vi "U3 DAC Function Generator.vi"() -> ()   [LabVIEW 2010]
panel:
  out "Error":string
  in  "Min Voltage":dbl=0.5 min=0.0 max=5.0 step=0.1 format="%.2f"
  in  "Stop":bool
  # "SMT Signal Cluster (complexl).ctlUpdates DAC0 at the specified update interval in order to build time series waveforms.  The\nupdate interval is set to 20 ms by default, but can be set lower based on the execution times\ndiscussed in Section 3.1 of the U3 User's Guide.  Uses the first found U3.\n\nWith a software timed application such as this, you might be able to reduce timing jitter (caused\nby the operating system) by increasing the priority of this process (labview.exe) in Windows\nTask Manager."
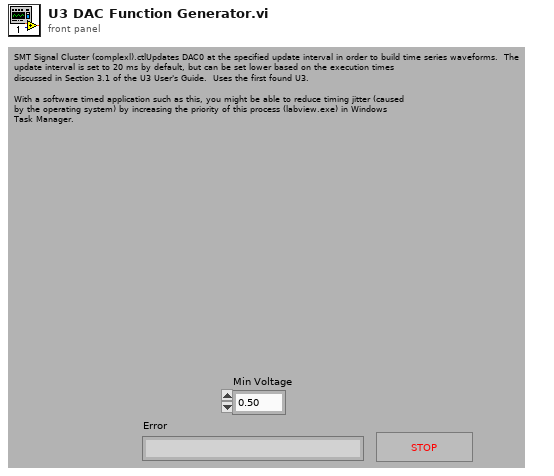
[diagram p1: front panel]
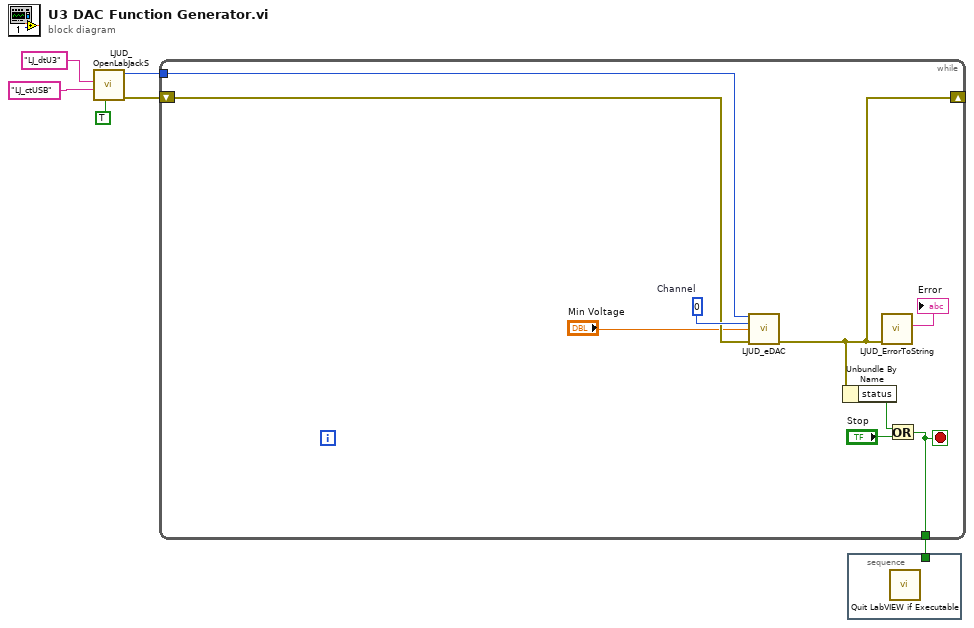
[diagram p0: block diagram]
diagram:
  n1 = call "LJUD_OpenLabJackS.vi"("FirstFound"=TRUE, "ConnectionType"="LJ_ctUSB", "DeviceType"="LJ_dtU3") -> ("error out"=w2:errorcluster, "Handle"=w1:i32)  [unwired: 6 in, 1 out]
  n2 = while {
    tunnel: w1 -> [w8]
    shift-left: w2 -> [w10]
    shift-right: [w9] -> _
    tunnel: [w12] -> w6
    stop <- w12 stop-if-true
    w11 = 0  # Channel
    n3 = call "LJUD_eDAC.vi"("Handle In"=w8, "Channel"=w11, "Voltage"="Min Voltage", "error in"=w10) -> ("error out"=w9:errorcluster)  [unwired: 10 in, 1 out]
    n4 = Unbundle By Name(w9) -> ("status"=w13:bool)
    n5 = call "LJUD_ErrorToString.vi"("error in"=w9) -> ("String"=→"Error":string)  [unwired: 10 in]
    n6 = Or(x=w13, y="Stop") -> (x .or. y?=w12:bool)
  }
  n7 = stacked-sequence {
    tunnel: w6 -> [_]
    frame #0 {
      n8 = call "Quit LabVIEW if Executable.vi"() -> ()  [unwired: 1 in]
    }
  }
